vi "List Contained Messages.vi"(8 "error in (no error)":errorcluster, 11 "Message":refnum<class "Message.lvclass">) -> (0 "error out":errorcluster, 3 "Message Array":refnum<class "Message.lvclass">[](array[class]))   [LabVIEW 2020, in "Sequencer.lvlib"]
doc: "Recursivly get all messages nested in 'Message'."
uses:
  Sequencer.lvlib
  PPL/HDH.Actor Framework.Core.Actor.lvlibp/1abvi3w/vi.lib/ActorFramework/Message/Message.lvclass
  Sequencer Messages/Batch Msg/Batch Msg.lvclass
  C:/Current projects/WS/PPL/HDH.Actor Framework.Core.Actor.lvlibp/1abvi3w/vi.lib/ActorFramework/Message/Message.lvclass
  Sequencer Messages/Batch Msg/Batch Msg.lvclass/Batch Msg.ctl
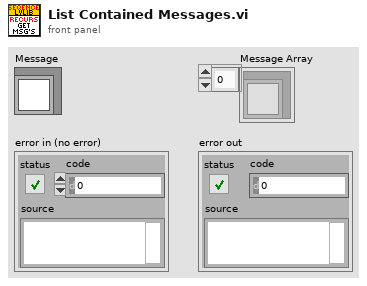
[diagram p1: front panel]
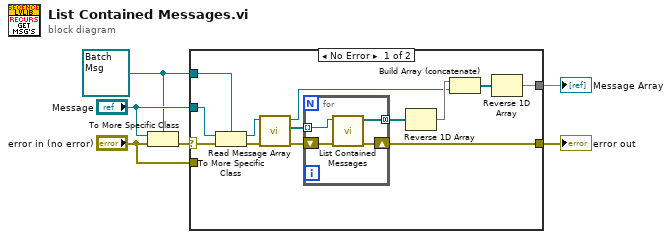
[diagram p0: block diagram]
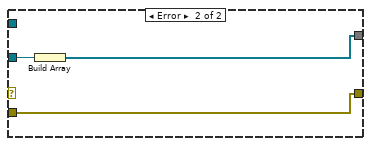
[diagram p2: hidden frame]
diagram:
  w1 = refnum<class "Batch Msg.lvclass"> refnum ("Sequencer.lvlib:Batch Msg.lvclass")
  n1 = To More Specific Class(target class=w1, reference="Message", error in="error in (no error)") -> (error out=w6:errorcluster)  [unwired: 1 out]
  n2 = case shown="No Error" w6 {
    selector: w6 -> [w19 _]
    tunnel: "Message" -> [w18 w26]
    tunnel: [w8 w25] -> w4
    tunnel: [w7 w24] -> w3
    tunnel: "error in (no error)" -> [_ w24]
    tunnel: w1 -> [w17 _]
    frame No Error {
      n3 = To More Specific Class(target class=w17, reference=w18, error in=w19) -> (specific class reference=w16:refnum<class "Batch Msg.lvclass">, error out=w15:errorcluster)
      n4 = call "Read Message Array.vi"("error in (no error)"=w15, "Batch Msg in"=w16) -> ("error out"=w13:errorcluster, "Message Array"=w14:refnum<class "Message.lvclass">[], "Batch Msg out"=w10:refnum<class "Batch Msg.lvclass">)  [unwired: 7 in]
      n5 = for {
        tunnel: w14 -> [w23] mode=indexing
        shift-right: [w21] -> w7
        shift-left: w13 -> [w22]
        tunnel: [w20] -> w12 mode=concatenating
        n6 = call "List Contained Messages.vi"("error in (no error)"=w22, "Message"=w23) -> ("error out"=w21:errorcluster, "Message Array"=w20:refnum<class "Message.lvclass">[])  [unwired: 8 in]
      }
      n7 = Reverse 1D Array(array=w12) -> (reversed array=w11:refnum<class "Message.lvclass">[])
      n8 = Build Array (concatenate)(w11, w10) -> (w9:refnum<class "Message.lvclass">[])
      n9 = Reverse 1D Array(array=w9) -> (reversed array=w8:refnum<class "Message.lvclass">[])
    }
    frame Error {
      n10 = Build Array(w26) -> (w25:refnum<class "Message.lvclass">[])
    }
  }
  "error out" <- w3
  "Message Array" <- w4
